vi "Configure Session.vi"(4 "serialCfg":T1={"baud rate (9600)"=9600, "data bits (8)"=7, "stop bits (10: 1 bit)"=10, "parity (0:none)"=enum."Even", "flow control (0:none)"=0, "endModeforReads"=2, "endModeforWrites"=2} {"stop bits (10: 1 bit)" items=["1.0"=10, "1.5"=15, "2.0"=20]; "flow control (0:none)" items=["None", "XON/XOFF", "RTS/CTS", "XON/XOFF & RTS/CTS", "DTR/DSR", "XON/XOFF & DTR/DSR"]; "endModeforReads" items=["None", "Last Bit", "TermChar"]; "endModeforWrites" items=["None", "Last Bit", "TermChar", "Break"]}, 6 "Message Cfg":T2={"EnTermChar"=TRUE, "termChar"=13, "suppEnEnRd"=FALSE, "sendEndEn"=TRUE}, 7 "timeout":u32=100, 8 "error in":errorcluster, 10 "VISA Resource":refnum<visa-resource-name>, 11 "Serial Session":refnum<class "Serial Session.lvclass">) -> (0 "error out":errorcluster, 3 "Serial Session out":refnum<class "Serial Session.lvclass">)   [LabVIEW 2019, in "Serial Session.lvclass"]
doc: "Configures a session using the VISA serial property nodes. Call this before opening any references to the session. After this, the ESF will handle all calls to the port via the session handle."
uses:
  Serial Session.lvclass
  Serial Session.lvclass/Serial Session.ctl
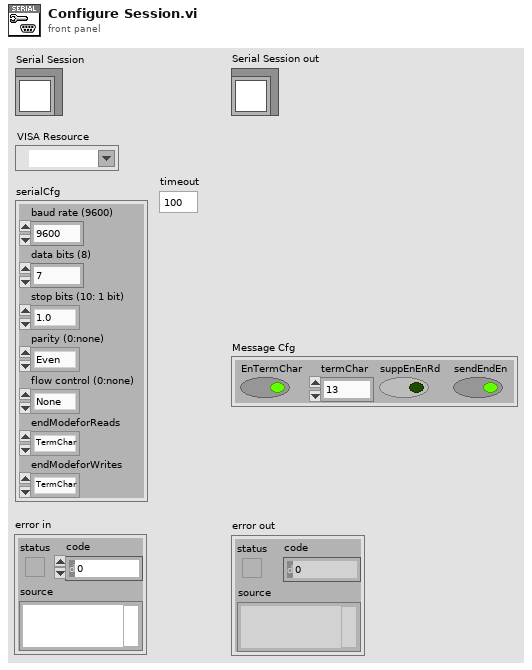
[diagram p1: front panel]
types:
  T1 = cluster{"baud rate (9600)":u32, "data bits (8)":u16, "stop bits (10: 1 bit)":u16, "parity (0:none)":enum16{"None", "Odd", "Even", "Mark", "Space"}, "flow control (0:none)":u16, "endModeforReads":u16, "endModeforWrites":u16}
  T2 = cluster{"EnTermChar":bool, "termChar":u8, "suppEnEnRd":bool, "sendEndEn":bool}
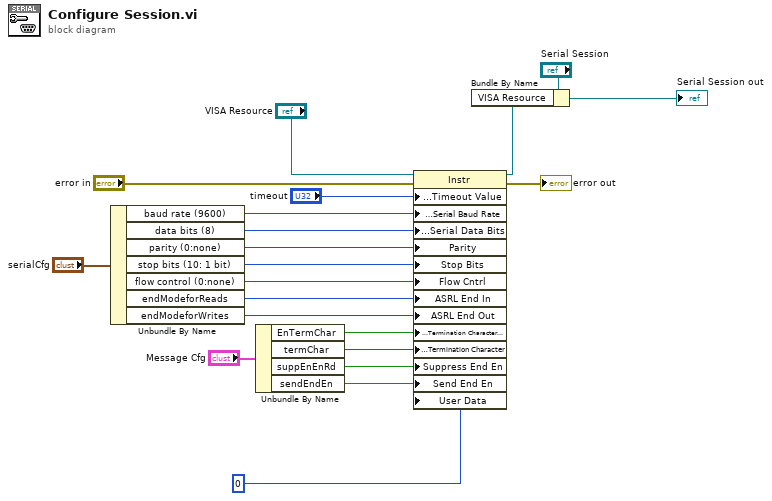
[diagram p0: block diagram]
diagram:
  n1 = Unbundle By Name("serialCfg") -> ("baud rate (9600)"=w20:u32, "data bits (8)"=w19:u16, "parity (0:none)"=w18:enum16{"None", "Odd", "Even", "Mark", "Space"}, "stop bits (10: 1 bit)"=w17:u16, "flow control (0:none)"=w16:u16, "endModeforReads"=w15:u16, "endModeforWrites"=w14:u16)
  n2 = Unbundle By Name("Message Cfg") -> ("EnTermChar"=w13:bool, "termChar"=w12:u8, "suppEnEnRd"=w11:bool, "sendEndEn"=w10:bool)
  n3 = property class="Instr"(reference="VISA Resource", error in="error in", "General Settings:Timeout Value"="timeout", "Serial Settings:Serial Baud Rate"=w20, "Serial Settings:Serial Data Bits"=w19, "Parity"=w18, "Stop Bits"=w17, "Flow Cntrl"=w16, "ASRL End In"=w15, "ASRL End Out"=w14, "Message Based Settings:Termination Character Enable"=w13, "Message Based Settings:Termination Character"=w12, "Suppress End En"=w11, "Send End En"=w10, "User Data"=u32 0 ("General Settings:User Data")) -> (reference out=w7:refnum<visa-resource-name>, error out=→"error out":errorcluster)
  n4 = Bundle By Name(cluster="Serial Session", "VISA Resource"=w7) -> (→"Serial Session out":refnum<class "Serial Session.lvclass">)
